vi "Wait phase sensor.vi"(8 "error in (no error)":errorcluster, 9 "Sensitivity time (ms)":u32, 10 "Phase sensor number":i32, 11 "Sense T/F":bool=TRUE) -> (0 "error IO":errorcluster)   [LabVIEW 2017]
panel:
  out "Stop":bool
  out "Signal":bool
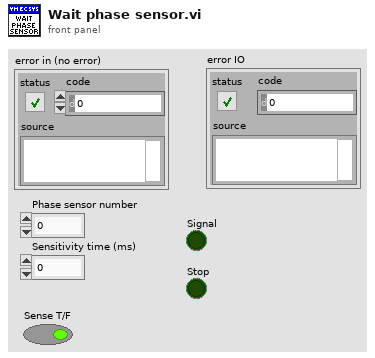
[diagram p1: front panel]
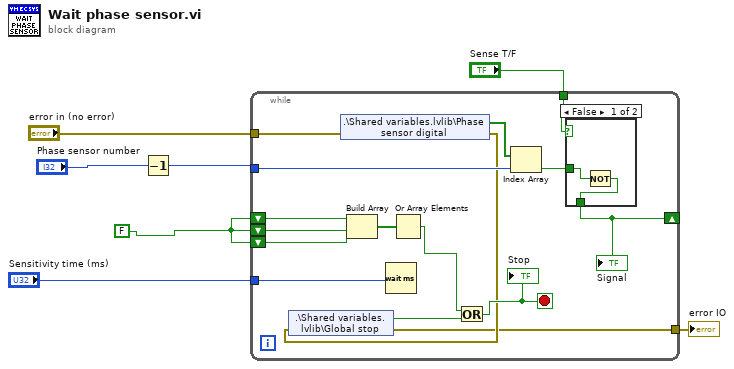
[diagram p0: block diagram]
diagram:
  w3 = FALSE ("Boolean")
  n1 = Decrement(x="Phase sensor number") -> (x-1=w7:i32)
  n2 = while {
    shift-right: [w8] -> _
    shift-left: w3 -> [w22]
    shift-left: w3 -> [w21]
    shift-left: w3 -> [w20]
    tunnel: w7 -> [w15]
    tunnel: "Sensitivity time (ms)" -> [w14]
    tunnel: "error in (no error)" -> [w13]
    tunnel: "Sense T/F" -> [w10]
    tunnel: [w11] -> w1
    stop <- w18 stop-if-true
    n3 = shared-variable ".\\Shared variables.lvlib\\Phase sensor digital"(error in=w13) -> (w23:bool[], error out=w12:errorcluster)
    n4 = shared-variable ".\\Shared variables.lvlib\\Global stop"(error in=w12) -> (w17:bool, error out=w11:errorcluster)
    n5 = Build Array(w22, w21, w20) -> (w19:bool[])
    n6 = Wait (ms)(milliseconds to wait=w14) -> ()  [unwired: 1 out]
    n7 = Or Array Elements(Boolean array=w19) -> (logical OR=w16:bool)
    n8 = Or(x=w16, y=w17) -> (x .or. y?=w18:bool)
    "Stop" <- w18
    n9 = Index Array(array=w23, index=w15) -> (element=w9:bool)
    n10 = case shown="False" w10 {
      tunnel: w9 -> [w25 w26]
      tunnel: [w24 w26] -> w8
      frame False {
        n11 = Not(x=w25) -> (.not. x?=w24:bool)
      }
      frame True {
      }
    }
    "Signal" <- w8
  }
  "error IO" <- w1
